vi "9_24_Fxp_addation.vi"(1 "y":fxp<+/-,24,9>, 2 "x":fxp<+/-,24,9>) -> (0 "x+y":fxp<+/-,25,10> format="%.41g")   [LabVIEW 2020]
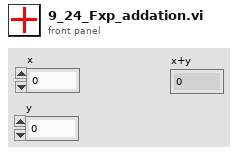
[diagram p1: front panel]
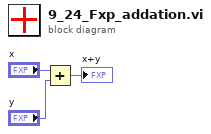
[diagram p0: block diagram]
diagram:
  n1 = Add(x="x", y="y") -> (x+y=→"x+y":fxp<+/-,25,10>)
